vi "Remove Channel by Name.vi"(8 "error in (no error)":errorcluster, 10 "Channel Name":string, 11 "CIFChannelMng in":refnum<class "CIFChannelMng.lvclass">) -> (0 "error out":errorcluster, 3 "CIFChannelMng out":refnum<class "CIFChannelMng.lvclass">)   [LabVIEW 2021, in "CIFChannelMng.lvclass"]
uses:
  CIFChannelMng.lvclass
  CIFChannelMng.lvclass/CIFChannelMng.ctl
  CIFChannels/CIFChannels.lvclass/CIFChannels.ctl
  CIFUtilities/CIFClocks/SubVIs/Add Error.vi
  CIFChannels/Accessors/Read Name.vi
  CIFChannels/Accessors/Write Channel State.vi
  CIFCore/Common/Utilities/Append Error Location.vi
  CIFChannels/CIFChannels.lvclass
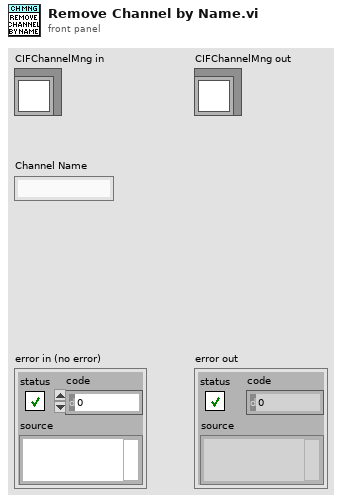
[diagram p1: front panel]
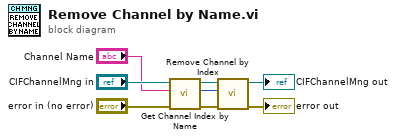
[diagram p0: block diagram]
diagram:
  n1 = call "Get Channel Index by Name.vi"("error in (no error)"="error in (no error)", "Channel Name"="Channel Name", "CIFChannelMng in"="CIFChannelMng in") -> ("error out"=w1:errorcluster, "Channel Index"=w2:i32, "CIFChannelMng out"=w3:refnum<class "CIFChannelMng.lvclass">)  [unwired: 6 in]
  n2 = call "Remove Channel by Index.vi"("error in (no error)"=w1, "Channel Index"=w2, "CIFChannelMng in"=w3) -> ("error out"=→"error out":errorcluster, "CIFChannelMng out"=→"CIFChannelMng out":refnum<class "CIFChannelMng.lvclass">)  [unwired: 7 in]
